vi "Perform Step.vi"(8 "error in (no error)":errorcluster, 11 "Window Action in":refnum<class "Window Action.lvclass">) -> (0 "error out":errorcluster, 2 "Result":T1, 3 "Window Action out":refnum<class "Window Action.lvclass">)   [LabVIEW 2020, in "MacroAssert.lvlib" / "Window Action.lvclass"]
doc: "Performs all actions required for <B>Step in</B>."
uses:
  Window Action.lvclass
  C:/Users/User/Documents/LabVIEW Data/Projects/MacroAssert/source/Classes/Step/Step.lvclass
  CTLs/Report Data.ctl
  9ebebc49-af8f-4fe3-a1a4-72e5e553d813.vi
  SubVIs/Win Util/Win Util.lvlib
  MacroAssert.lvlib
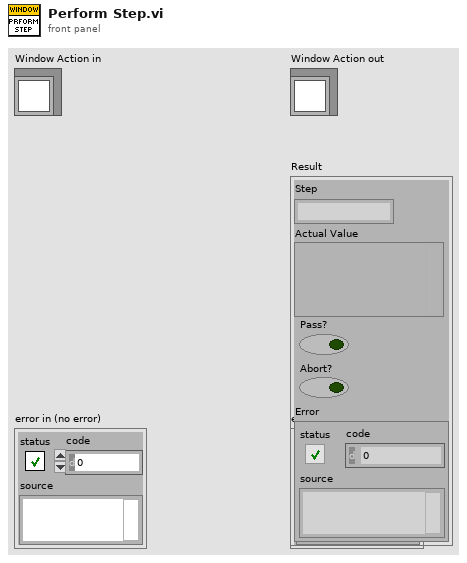
[diagram p1: front panel]
types:
  T1 = typedef "MacroAssert.lvlib/Report Data.ctl" = cluster{"Step":string, "Actual Value":variant, "Pass?":bool, "Abort?":bool, "Error":errorcluster}
  T2 = typedef "MacroAssert.lvlib/Window Action.lvclass/Window Action Type.ctl" = enum16{"Maximize Window", "Restore Window", "Minimize Window", "Close Window", "Bring Window to Front", "Send Window to Back"}
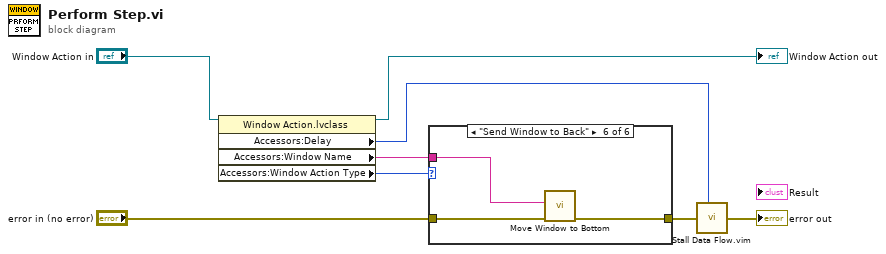
[diagram p0: block diagram]
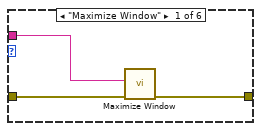
[diagram p2: hidden frame]
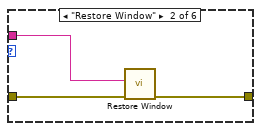
[diagram p3: hidden frame]
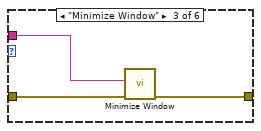
[diagram p4: hidden frame]
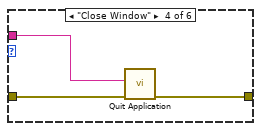
[diagram p5: hidden frame]
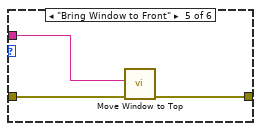
[diagram p6: hidden frame]
diagram:
  n1 = property class="Window Action.lvclass"(reference="Window Action in") -> (reference out=→"Window Action out":refnum<class "Window Action.lvclass">, "Accessors:Delay"=w1:i32, "Accessors:Window Name"=w5:string, "Accessors:Window Action Type"=w2:T2)  [unwired: 1 in, 1 out]
  n2 = case shown="\"Send Window to Back\"" w2 {
    tunnel: [w11 w14 w17 w20 w23 w26] -> w4
    tunnel: w5 -> [w10 w13 w16 w19 w22 w25]
    tunnel: "error in (no error)" -> [w9 w12 w15 w18 w21 w24]
    frame "Maximize Window" {
      n3 = call "Maximize Window.vi"("error in"=w9, "window name (\"\")"=w10) -> ("error out"=w11:errorcluster)  [unwired: 8 in, 1 out]
    }
    frame "Restore Window" {
      n4 = call "Restore Window.vi"("error in"=w12, "window name (\"\")"=w13) -> ("error out"=w14:errorcluster)  [unwired: 8 in, 1 out]
    }
    frame "Minimize Window" {
      n5 = call "Minimize Window.vi"("error in"=w15, "window name (\"\")"=w16) -> ("error out"=w17:errorcluster)  [unwired: 8 in, 1 out]
    }
    frame "Close Window" {
      n6 = call "Quit Application.vi"("error in (no error)"=w18, "window name (\"\")"=w19) -> ("error out"=w20:errorcluster)  [unwired: 9 in]
    }
    frame "Bring Window to Front" {
      n7 = call "Move Window to Top.vi"("error in"=w21, "window name (\"\")"=w22) -> ("error out"=w23:errorcluster)  [unwired: 8 in, 1 out]
    }
    frame "Send Window to Back" {
      n8 = call "Move Window to Bottom.vi"("error in"=w24, "window name (\"\")"=w25) -> ("error out"=w26:errorcluster)  [unwired: 8 in, 1 out]
    }
  }
  n9 = call "Stall Data Flow.vim"("value in"=w4, "milliseconds to wait"=w1) -> ("value out"=→"error out":errorcluster)  [unwired: 1 out]
